vi "TestExec.Add New SW Items to List, Overwrite if is existing.vi"(9 "New SW Items":T1[](array[typedef]), 11 "SW Items List":T1[](array[typedef])) -> (3 "SW Items List Out":T1[](array[typedef]))   [LabVIEW 2024]
uses:
  Results/Result XML/TestResult.SW Item.ctl
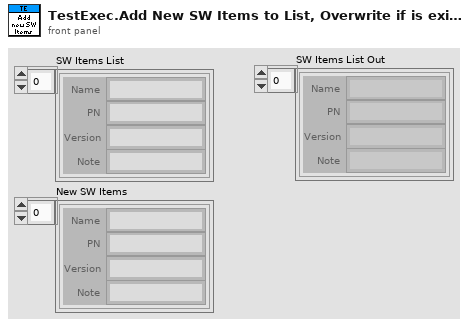
[diagram p1: front panel]
types:
  T1 = typedef "TestResult.SW Item.ctl" = cluster{"Name":string, "PN":string, "Version":string, "Note":string}
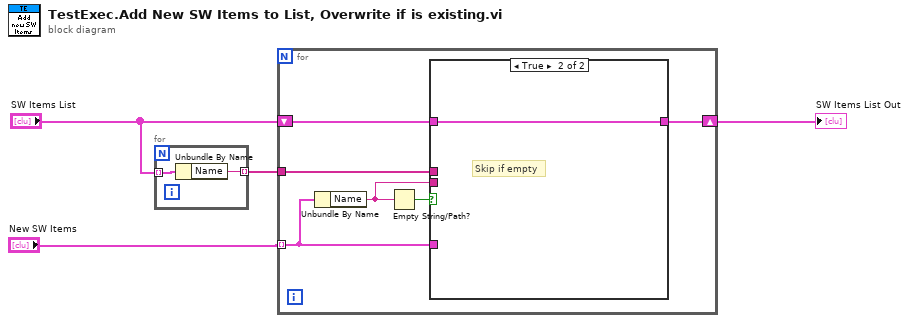
[diagram p0: block diagram]
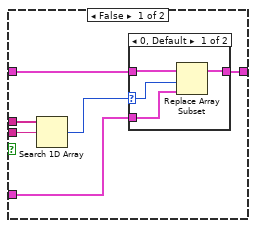
[diagram p2: hidden frame]
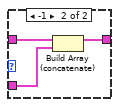
[diagram p3: hidden frame]
diagram:
  n1 = for {
    tunnel: "SW Items List" -> [w6] mode=indexing
    tunnel: [w5] -> w4 mode=indexing
    n2 = Unbundle By Name(w6) -> ("Name"=w5:string)
  }
  n3 = for {
    tunnel: "New SW Items" -> [w9] mode=indexing
    shift-right: [w11] -> w1
    shift-left: "SW Items List" -> [w12]
    tunnel: w4 -> [w10]
    n4 = Unbundle By Name(w9) -> ("Name"=w8:string)
    n5 = Empty String/Path?(string/path=w8) -> (empty?=w7:bool)
    n6 = case shown="True" w7 {
      tunnel: w12 -> [w18 w26]
      tunnel: [w17 w26] -> w11
      tunnel: w10 -> [w15 _]
      tunnel: w9 -> [w14 _]
      tunnel: w8 -> [w13 _]
      frame False {
        n7 = Search 1D Array(1D array=w15, element=w13) -> (index of element=w16:i32)  [unwired: 1 in]
        n8 = case shown="0, Default" w16 {
          selector: w16 -> [w19 _]
          tunnel: w18 -> [w22 w25]
          tunnel: [w21 w24] -> w17
          tunnel: w14 -> [w20 w23]
          frame 0, Default {
            n9 = Replace Array Subset(array=w22, new element=w20, index=w19) -> (w21:T1[])
          }
          frame -1 {
            n10 = Build Array (concatenate)(w25, w23) -> (w24:T1[])
          }
        }
      }
      frame True {
        # "Skip if empty"
      }
    }
  }
  "SW Items List Out" <- w1
